vi "Time_to_elapse.vi"() -> ()   [LabVIEW 2020]
doc: "Przechowuje czas, który musi odczekaæ timer."
panel:
  out "Numeric":dbl
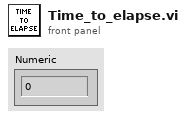
[diagram p1: front panel]
diagram:
